vi "MULTTCP2_BlockingServer.vi"(0 "stot ref":refnum<vi>, 1 "cmdset":string, 2 "block notifier":refnum<notifier>, 3 "blockID":string, 4 "blockport":u16, 5 "cmdq":string) -> ()   [LabVIEW 2016]
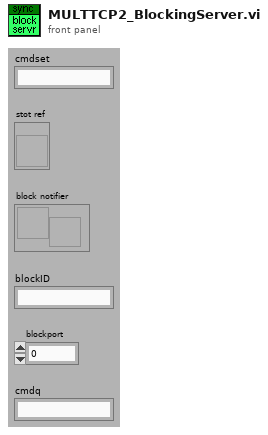
[diagram p1: front panel]
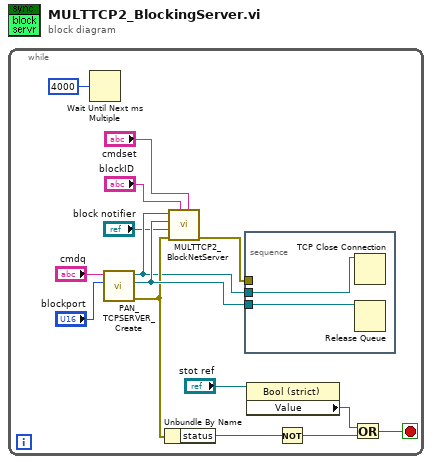
[diagram p0: block diagram]
diagram:
  n1 = while {
    stop <- w14 stop-if-true
    n2 = Wait Until Next ms Multiple(millisecond multiple=u32 4000) -> ()  [unwired: 1 out]
    n3 = call "PAN_TCPSERVER_Create.vi"("port"="blockport", "messages from socks Q name"="cmdq") -> ("error out"=w9:errorcluster, "queue out"=w10:refnum<queue>, "listener ID"=w7:refnum<k5>)  [unwired: 3 in, 4 out]
    n4 = Unbundle By Name(w9) -> ("status"=w11:bool)
    n5 = call "MULTTCP2_BlockNetServer.vi"("cmdset"="cmdset", "ID"="blockID", "error in (no error)"=w9, "notifier In"="block notifier", "messages from sock"=w10, "listener ID"=w7) -> ("error out"=w8:errorcluster)  [unwired: 5 out]
    n6 = stacked-sequence {
      tunnel: w10 -> [w17]
      tunnel: w8 -> [_]
      tunnel: w7 -> [w16]
      frame #0 {
        n7 = TCP Close Connection(connection ID=w16) -> ()  [unwired: 1 in, 3 out]
        n8 = Release Queue(queue=w17) -> ()  [unwired: 1 in, 4 out]
      }
    }
    n9 = property class="Bool (strict)"(reference="stot ref") -> ("Value"=w12:bool)  [unwired: 1 in, 2 out]
    n10 = Not(x=w11) -> (.not. x?=w13:bool)
    n11 = Or(x=w12, y=w13) -> (x .or. y?=w14:bool)
  }
